vi "IonHeating_wrapper.vi"(0 "Strings in":string[](array[string])=["C:\\CuspControl\\GPIB and Network\\Cusp\\AgilentName.txt", "6723"], 1 "Dubs in":dbl[](array[numeric])=[0.0, 12000.0, 15000.0, 0.011, 0.2]) -> ()   [LabVIEW 2018]
uses:
  <vilib>/DAQmx/write.llb/DAQmx Write (Analog DBL 1Chan 1Samp).vi
  <vilib>/DAQmx/create/channels.llb/DAQmx Create Channel (AO-Voltage-Basic).vi
  <vilib>/DAQmx/miscellaneous.llb/DAQmx Fill In Error Info.vi
panel:
  out "error out":errorcluster
  in  "relay ao line":string="/ao3"
  in  "AO2 name":string="6723"
  out "IH on":bool
  in  "IH setgs":T1={"Start Frequency"=12000.0, "Stop Frequency"=15000.0, "Sweep Time"=0.011, "Amplitude"=0.2} {"Sweep Time" format="%.4f"; "Stop Frequency" format="%^.5e"; "Start Frequency" format="%^.5e"; "Amplitude" min=0.0 max=4.0 format="%.3f"}
  out "VISAsession":string="agi33522a"
  in  "Synth name file":path=path "C:/CuspControl/GPIB and Network/Cusp/AgilentName.txt"
  in  "subvi":bool=TRUE
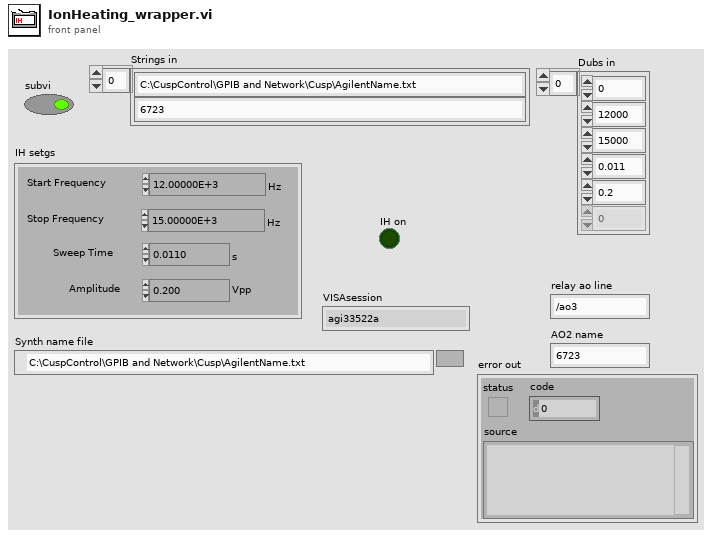
[diagram p1: front panel]
types:
  T1 = cluster{"Start Frequency":dbl, "Stop Frequency":dbl, "Sweep Time":dbl, "Amplitude":dbl}
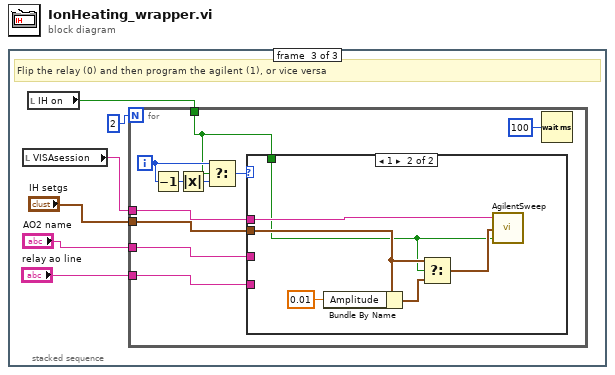
[diagram p0: block diagram]
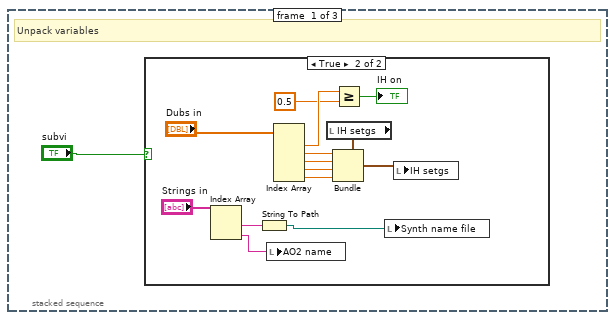
[diagram p2: hidden frame]
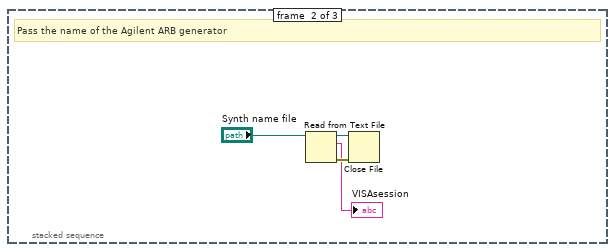
[diagram p4: hidden frame]
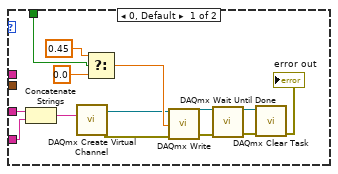
[diagram p5: hidden frame]
diagram:
  n1 = stacked-sequence {
    frame #0 {
      # "Unpack variables"
      n2 = case shown="True" "subvi" {
        frame False {
        }
        frame True {
          n3 = Index Array(array="Strings in") -> (element #1=w14:string, element #2=w2:string)  [unwired: 2 in]
          n4 = String To Path(string=w14) -> (path=w13:path)
          n5 = local write "AO2 name"(w2) -> ()
          n6 = Index Array(array="Dubs in") -> (element #1=w9:dbl, element #2=w6:dbl, element #3=w5:dbl, element #4=w4:dbl, element #5=w3:dbl)  [unwired: 5 in]
          n7 = local read "IH setgs"() -> (w11:T1)
          n8 = Bundle(cluster=w11, "Start Frequency"=w6, "Stop Frequency"=w5, "Sweep Time"=w4, "Amplitude"=w3) -> (w10:T1)
          n9 = Greater Or Equal?(x=w9, y=0.5) -> (x >= y?=→"IH on":bool)
          n10 = local write "Synth name file"(w13) -> ()
          n11 = local write "IH setgs"(w10) -> ()
        }
      }
    }
    frame #1 {
      # "Pass the name of the Agilent ARB generator"
      n12 = Read from Text File(file (use dialog)="Synth name file") -> (refnum out=w17:refnum<file>, text=→"VISAsession":string, error out=w18:errorcluster)  [unwired: 3 in, 1 out]
      n13 = Close File(refnum=w17, error in=w18) -> ()  [unwired: 2 out]
    }
    frame #2 {
      # "Flip the relay (0) and then program the agilent (1), or vice versa"
      n14 = local read "VISAsession"() -> (w22:string)
      n15 = local read "IH on"() -> (w20:bool)
      n16 = for {
        N: 2 -> [_]
        tunnel: "relay ao line" -> [w35]
        tunnel: "AO2 name" -> [w34]
        tunnel: "IH setgs" -> [w33]
        tunnel: w22 -> [w32]
        tunnel: w20 -> [w27]
        i -> [w28]
        n17 = Decrement(x=w28) -> (x-1=w31:i32)
        n18 = Absolute Value(x=w31) -> (abs(x)=w30:i32)
        n19 = Select(t=w28, s=w27, f=w30) -> (s? t:f=w29:i32)
        n20 = case shown="1" w29 {
          tunnel: w35 -> [w49 _]
          tunnel: w34 -> [w48 _]
          tunnel: w27 -> [w38 w51]
          tunnel: w33 -> [_ w54]
          tunnel: w32 -> [_ w55]
          frame 0, Default {
            n21 = Concatenate Strings(w48, w49) -> (w37:string)
            n22 = call-poly <vilib>:"DAQmx Create Virtual Channel.vi"("physical channels"=w37) -> ("task out"=w39:refnum<k21>, "error out"=w40:errorcluster)  [unwired: 13 in]
            n23 = Select(t=0.45 ("ON voltage"), s=w38, f=0.0) -> (s? t:f=w46:dbl)
            n24 = call-poly <vilib>:"DAQmx Write.vi"("task/channels in"=w39, "data"=w46, "error in"=w40) -> ("task out"=w43:refnum<k21>, "error out"=w44:errorcluster)  [unwired: 10 in, 1 out]
            n25 = call <vilib>:"DAQmx Wait Until Done.vi"("task/channels in"=w43, "error in"=w44) -> ("task out"=w41:refnum<k21>, "error out"=w42:errorcluster)  [unwired: 12 in]
            n26 = call <vilib>:"DAQmx Clear Task.vi"("task in"=w41, "error in"=w42) -> ("error out"=→"error out":errorcluster)  [unwired: 13 in]
          }
          frame 1 {
            n27 = Bundle By Name(cluster=w54, "Amplitude"=0.01) -> (w53:T1)
            n28 = Select(t=w54, s=w51, f=w53) -> (s? t:f=w52:T1)
            n29 = call "AgilentSweep.vi"("Enable Output (T: Enable)"=w51, "IH setgs"=w52, "VISA resource name"=w55) -> ()
          }
        }
        n30 = Wait (ms)(milliseconds to wait=u32 100) -> ()  [unwired: 1 out]
      }
    }
  }
